vi "游标显示.vi"(0 "WaveformGraph输入":refnum<vi>, 1 "V2":dbl, 2 "tv":dbl, 3 "tv_end":dbl, 4 "V1":dbl, 5 "td2":dbl, 6 "tv_start":dbl, 7 "ts2":dbl, 8 "ts":dbl, 10 "td":dbl, 11 "I100%":dbl, 12 "ts1":dbl, 13 "I0%":dbl) -> ()   [LabVIEW 2011]
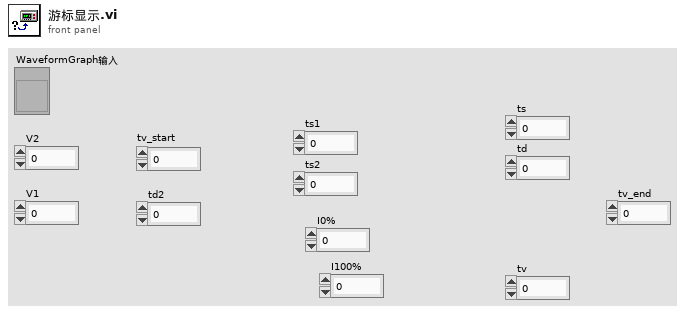
[diagram p1: front panel]
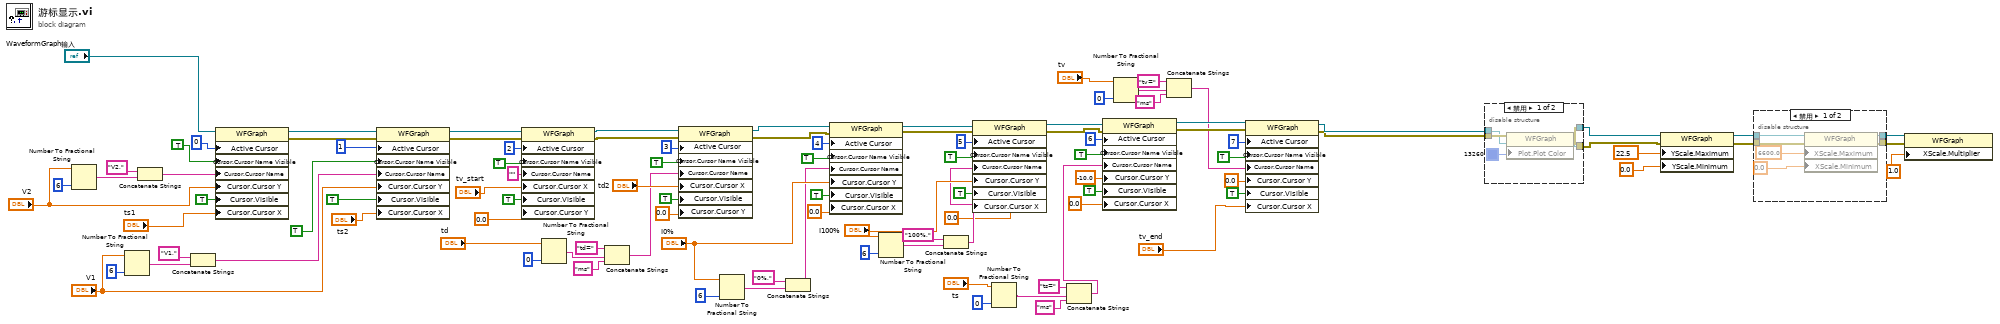
[diagram p0: block diagram]
diagram:
  n1 = Number To Fractional String(number="V2", precision (6)=i16 6 ("宽度(-)")) -> (F-format string=w89:string)  [unwired: 2 in]
  n2 = Number To Fractional String(number="V1", precision (6)=i16 6 ("宽度(-)")) -> (F-format string=w94:string)  [unwired: 2 in]
  n3 = Concatenate Strings("V2," ("光标.游标名"), w89) -> (w91:string)
  n4 = Concatenate Strings("V1," ("光标.游标名"), w94) -> (w92:string)
  n5 = property on="属性节点" class="WFGraph"(reference="WaveformGraph输入", "Active Cursor"=u32 0 ("活动游标"), "Cursor.Cursor Name Visible"=TRUE ("光标.游标名可见"), "Cursor.Cursor Name"=w91, "Cursor.Cursor Y"="V2", "Cursor.Visible"=TRUE ("光标.可见"), "Cursor.Cursor X"="ts1") -> (reference out=w26:refnum<vi>, error out=w100:errorcluster)  [unwired: 1 in]
  n6 = property on="属性节点" class="WFGraph"(reference=w26, error in=w100, "Active Cursor"=u32 1 ("活动游标"), "Cursor.Cursor Name Visible"=TRUE ("光标.游标名可见"), "Cursor.Cursor Name"=w92, "Cursor.Cursor Y"="V1", "Cursor.Visible"=TRUE ("光标.可见"), "Cursor.Cursor X"="ts2") -> (reference out=w84:refnum<vi>, error out=w83:errorcluster)
  n7 = property on="属性节点" class="WFGraph"(reference=w84, error in=w83, "Active Cursor"=u32 2 ("活动游标"), "Cursor.Cursor Name Visible"=TRUE ("光标.游标名可见"), "Cursor.Cursor Name"="" ("光标.游标名"), "Cursor.Cursor X"="tv_start", "Cursor.Visible"=TRUE ("光标.可见"), "Cursor.Cursor Y"=0.0 ("光标.游标位置:游标Y坐标")) -> (reference out=w75:refnum<vi>, error out=w74:errorcluster)
  n8 = Number To Fractional String(number="td", precision (6)=i16 0 ("宽度(-)")) -> (F-format string=w30:string)  [unwired: 2 in]
  n9 = Concatenate Strings("td=" ("字符串"), w30, "ms" ("字符串")) -> (w29:string)
  n10 = property on="属性节点" class="WFGraph"(reference=w75, error in=w74, "Active Cursor"=u32 3 ("活动游标"), "Cursor.Cursor Name Visible"=TRUE ("光标.游标名可见"), "Cursor.Cursor Name"=w29, "Cursor.Cursor X"="td2", "Cursor.Visible"=TRUE ("光标.可见"), "Cursor.Cursor Y"=0.0 ("光标.游标位置:游标Y坐标")) -> (reference out=w63:refnum<vi>, error out=w60:errorcluster)
  n11 = Number To Fractional String(number="I0%", precision (6)=i16 6 ("宽度(-)")) -> (F-format string=w52:string)  [unwired: 2 in]
  n12 = Concatenate Strings("0%," ("光标.游标名"), w52) -> (w49:string)
  n13 = property on="属性节点" class="WFGraph"(reference=w63, error in=w60, "Active Cursor"=u32 4 ("活动游标"), "Cursor.Cursor Name Visible"=TRUE ("光标.游标名可见"), "Cursor.Cursor Name"=w49, "Cursor.Cursor Y"="I0%", "Cursor.Visible"=TRUE ("光标.可见"), "Cursor.Cursor X"=0.0 ("光标.游标位置:游标X坐标")) -> (reference out=w62:refnum<vi>, error out=w61:errorcluster)
  n14 = Number To Fractional String(number="I100%", precision (6)=i16 6 ("宽度(-)")) -> (F-format string=w47:string)  [unwired: 2 in]
  n15 = Concatenate Strings("100%," ("光标.游标名"), w47) -> (w44:string)
  n16 = property on="属性节点" class="WFGraph"(reference=w62, error in=w61, "Active Cursor"=u32 5 ("活动游标"), "Cursor.Cursor Name Visible"=TRUE ("光标.游标名可见"), "Cursor.Cursor Name"=w44, "Cursor.Cursor Y"="I100%", "Cursor.Visible"=TRUE ("光标.可见"), "Cursor.Cursor X"=0.0 ("光标.游标位置:游标X坐标")) -> (reference out=w56:refnum<vi>, error out=w55:errorcluster)
  n17 = Number To Fractional String(number="ts", precision (6)=i16 0 ("宽度(-)")) -> (F-format string=w28:string)  [unwired: 2 in]
  n18 = Concatenate Strings("ts=" ("字符串"), w28, "ms" ("字符串")) -> (w27:string)
  n19 = property on="属性节点" class="WFGraph"(reference=w56, error in=w55, "Active Cursor"=u32 6 ("活动游标"), "Cursor.Cursor Name Visible"=TRUE ("光标.游标名可见"), "Cursor.Cursor Name"=w27, "Cursor.Cursor Y"=-10.0 ("光标.游标位置:游标Y坐标"), "Cursor.Visible"=TRUE ("光标.可见"), "Cursor.Cursor X"=0.0 ("光标.游标位置:游标X坐标")) -> (reference out=w9:refnum<vi>, error out=w8:errorcluster)
  n20 = Number To Fractional String(number="tv", precision (6)=i16 0 ("宽度(-)")) -> (F-format string=w37:string)  [unwired: 2 in]
  n21 = Concatenate Strings("tv=" ("字符串"), w37, "ms" ("字符串")) -> (w4:string)
  n22 = property on="属性节点" class="WFGraph"(reference=w9, error in=w8, "Active Cursor"=u32 7 ("活动游标"), "Cursor.Cursor Name Visible"=TRUE ("光标.游标名可见"), "Cursor.Cursor Name"=w4, "Cursor.Cursor Y"=0.0 ("光标.游标位置:游标Y坐标"), "Cursor.Visible"=TRUE ("光标.可见"), "Cursor.Cursor X"="tv_end") -> (reference out=w7:refnum<vi>, error out=w6:errorcluster)
  n23 = disable-structure shown="禁用" {
    disable-tunnel: [w106 w107] -> w3
    disable-tunnel: [w104 w108] -> w2
    disable-tunnel: w6 -> [w103 w108]
    disable-tunnel: w7 -> [w102 w107]
    frame Disabled {
      n24 = property on="属性节点" class="WFGraph"(reference=w103, error in=w102, "Plot.Plot Color"=u32 13260) -> (reference out=w104:refnum<vi>, error out=w106:errorcluster)
    }
    frame Enabled {
    }
  }
  n25 = property on="属性节点" class="WFGraph"(reference=w3, error in=w2, "YScale.Maximum"=22.5 ("Y标尺.范围:最大值"), "YScale.Minimum"=0.0 ("Y标尺.范围:最小值")) -> (reference out=w22:refnum<vi>, error out=w25:errorcluster)
  n26 = disable-structure shown="禁用" {
    disable-tunnel: w25 -> [w114 w115]
    disable-tunnel: w22 -> [w113 w116]
    disable-tunnel: [w110 w116] -> w21
    disable-tunnel: [w109 w115] -> w20
    frame Disabled {
      n27 = property on="属性节点" class="WFGraph"(reference=w113, error in=w114, "XScale.Maximum"=6600.0 ("X标尺.范围:最大值"), "XScale.Minimum"=0.0 ("X标尺.范围:最小值")) -> (reference out=w110:refnum<vi>, error out=w109:errorcluster)
    }
    frame Enabled {
    }
  }
  n28 = property on="属性节点" class="WFGraph"(reference=w21, error in=w20, "XScale.Multiplier"=1.0 ("X标尺.偏移量与缩放系数:缩放系数")) -> ()  [unwired: 2 out]
